vi "All User Roles.vi"(8 "error in (no error)":errorcluster, 11 "Security in":refnum<class "Security.lvclass">) -> (0 "error out":errorcluster, 2 "User Roles":string[](array[string]), 3 "Security out":refnum<class "Security.lvclass">)   [LabVIEW 2020, in "HTTP Server.lvlib" / "Security.lvclass"]
uses:
  Security.lvclass
  Security.lvclass/Security.ctl
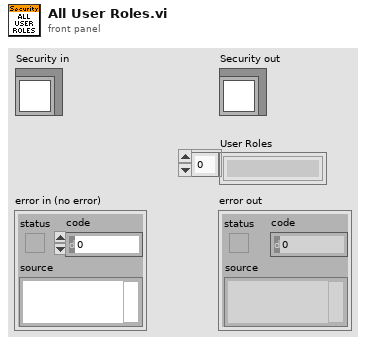
[diagram p1: front panel]
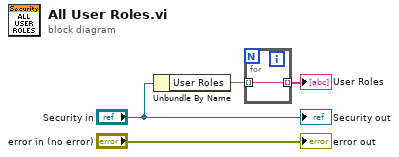
[diagram p0: block diagram]
diagram:
  n1 = Unbundle By Name("Security in") -> ("User Roles"=w2:set{string})
  n2 = for {
    tunnel: w2 -> [w5] mode=indexing
    tunnel: [w5] -> w1 mode=indexing
  }
  "User Roles" <- w1
  "error out" <- "error in (no error)"
  "Security out" <- "Security in"
